vi "Assignment7.vi"() -> ()   [LabVIEW 2021]
panel:
  in  "stop":bool
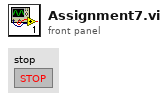
[diagram p1: front panel]
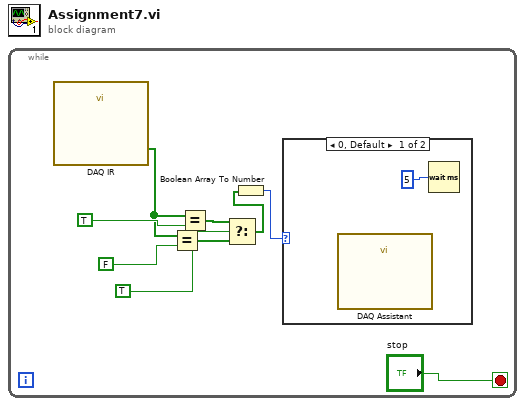
[diagram p0: block diagram]
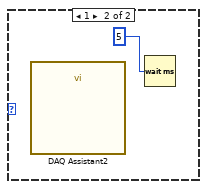
[diagram p2: hidden frame]
diagram:
  n1 = while {
    stop <- "stop" stop-if-true
    n2 = call "DAQ IR"() -> ("data"=w6:bool[])  [unwired: 17 in, 2 out]
    n3 = Equal?(x=w6, y=FALSE) -> (x = y?=w4:bool[])
    n4 = Equal?(x=w6, y=TRUE) -> (x = y?=w5:bool[])
    n5 = Select(t=w5, s=TRUE, f=w4) -> (s? t:f=w1:bool[])
    n6 = Boolean Array To Number(Boolean array=w1) -> (number=w2:u32)
    n7 = case shown="0, Default" w2 {
      frame 0, Default {
        n8 = call "DAQ Assistant"() -> ()  [unwired: 18 in, 2 out]
        n9 = Wait (ms)(milliseconds to wait=u32 5) -> ()  [unwired: 1 out]
      }
      frame 1 {
        n10 = call "DAQ Assistant2"() -> ()  [unwired: 18 in, 2 out]
        n11 = Wait (ms)(milliseconds to wait=u32 5) -> ()  [unwired: 1 out]
      }
    }
  }
